vi "Get Top Controls.vi"(11 "vi path":path=path "C:/Users/lubo/Documents/LabView/LabVIEW-Universal-Transcriptor/Test/Example Test 1.vi") -> (2 "Count of controls of specified datatype":i32, 3 "Controls Referencies Array":refnum<vi>[](array[refnum]))   [LabVIEW 2014]
panel:
  in  "DataType":string(combo)="error"
  # "This example returns count of controls of specified datatype, ie. if we\nchoose double, it returns count of controls at top level in VI of type\n'double'"
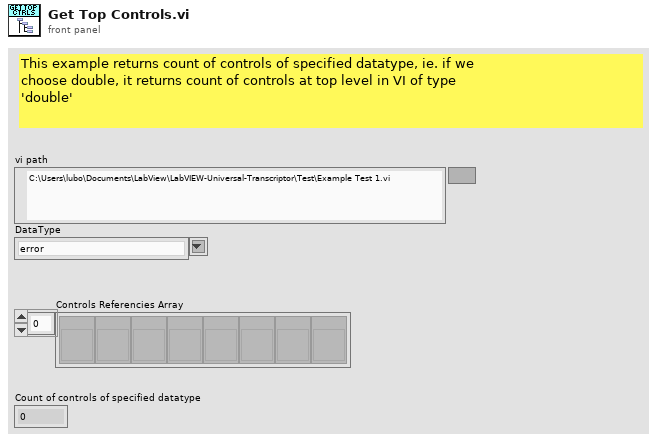
[diagram p1: front panel]
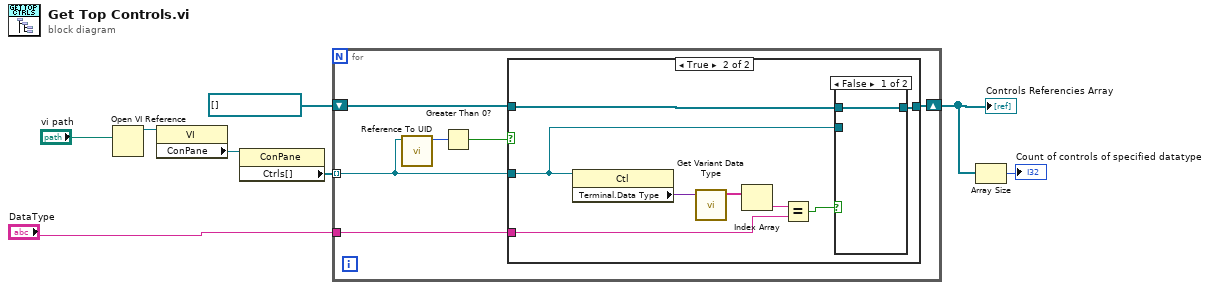
[diagram p0: block diagram]
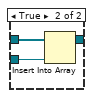
[diagram p3: hidden frame]
diagram:
  n1 = Open VI Reference(vi path="vi path") -> (vi reference=w7:refnum<vi>)  [unwired: 5 in, 1 out]
  n2 = property class="VI"(reference=w7) -> ("ConPane"=w8:refnum<vi>)  [unwired: 1 in, 2 out]
  n3 = property class="ConPane"(reference=w8) -> ("Ctrls[]"=w6:refnum<vi>[])  [unwired: 1 in, 2 out]
  n4 = for {
    tunnel: w6 -> [w11] mode=indexing
    tunnel: "DataType" -> [w14]
    shift-right: [w12] -> w3
    shift-left: refnum<vi>[] [] -> [w13]
    n5 = call "Reference To UID.vi"("Reference"=w11) -> ("UID"=w10:i32)  [unwired: 10 in]
    n6 = Greater Than 0?(x=w10) -> (x > 0?=w9:bool)
    n7 = case shown="True" w9 {
      tunnel: w14 -> [_ w20]
      tunnel: w13 -> [w15 w18]
      tunnel: w11 -> [_ w17]
      tunnel: [w15 w16] -> w12
      frame False {
      }
      frame True {
        n8 = property class="Ctl"(reference=w17) -> ("Terminal.Data Type"=w23:variant)  [unwired: 1 in, 2 out]
        n9 = call "Get Variant Data Type.vi"("variant"=w23) -> ("Data Type"=w22:string[])  [unwired: 10 in]
        n10 = Index Array(array=w22) -> (element=w21:string)  [unwired: 1 in]
        n11 = Equal?(x=w21, y=w20) -> (x = y?=w19:bool)
        n12 = case shown="False" w19 {
          tunnel: w18 -> [w24 w27]
          tunnel: w17 -> [_ w26]
          tunnel: [w24 w25] -> w16
          frame False {
          }
          frame True {
            n13 = Insert Into Array(array=w27, new element=w26) -> (w25:refnum<vi>[])  [unwired: 1 in]
          }
        }
      }
    }
  }
  "Controls Referencies Array" <- w3
  n14 = Array Size(array=w3) -> (size(s)=→"Count of controls of specified datatype":i32)
